vi "Sort Balls.vi"(11 "Detection Ball \nArray":T1[](array[typedef])) -> (3 "Sorted Detection Ball \nArray":T1[](array[typedef]))   [LabVIEW 2018]
uses:
  SSL Detection Ball.ctl
  <vilib>/Analysis/Matrix/Datatypes/RealMatrix.ctl
  <vilib>/Analysis/Matrix/NI_Matrix.lvlib
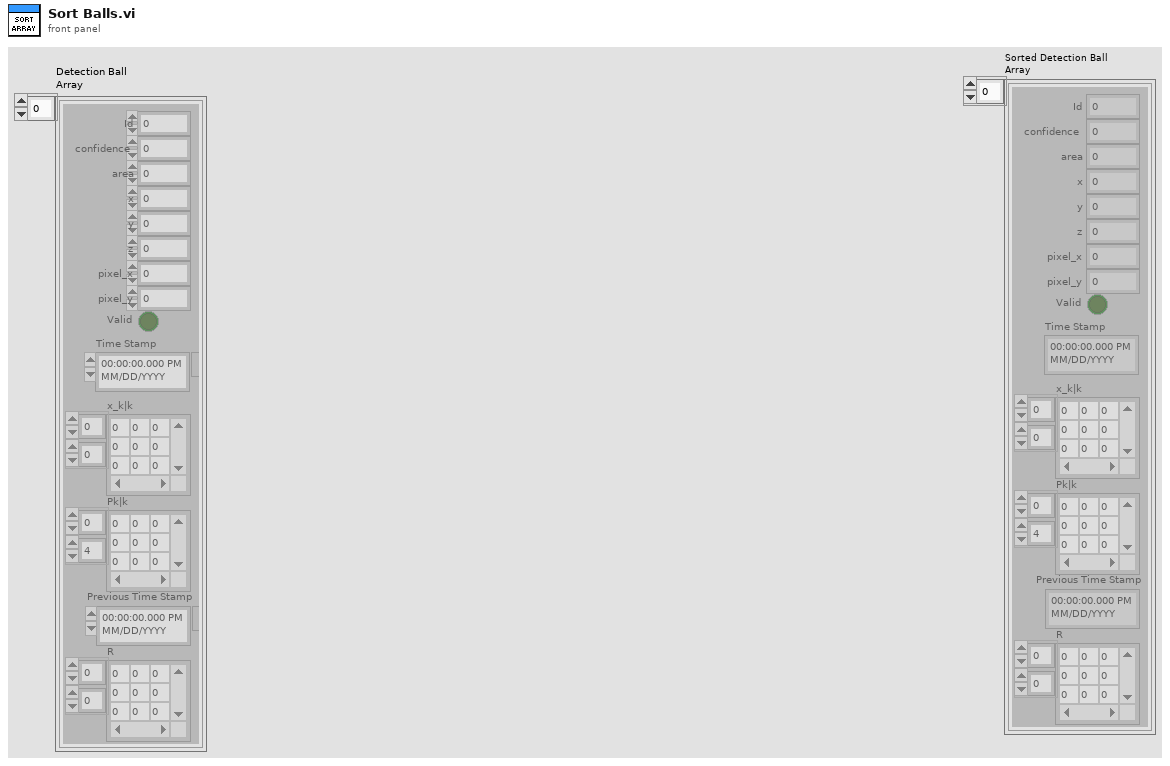
[diagram p1: front panel]
types:
  T1 = typedef "SSL Detection Ball.ctl" = cluster{"x":sgl, "area":u32, "confidence":sgl, "y":sgl, "z":sgl, "pixel_x":sgl, "pixel_y":sgl, "Valid":bool, "Time Stamp":timestamp, "x_k|k":T2, "Pk|k":T2, "Id":u32, "Previous Time Stamp":timestamp, "R":T2}
  T2 = typedef "NI_Matrix.lvlib/RealMatrix.ctl" = dbl[][]
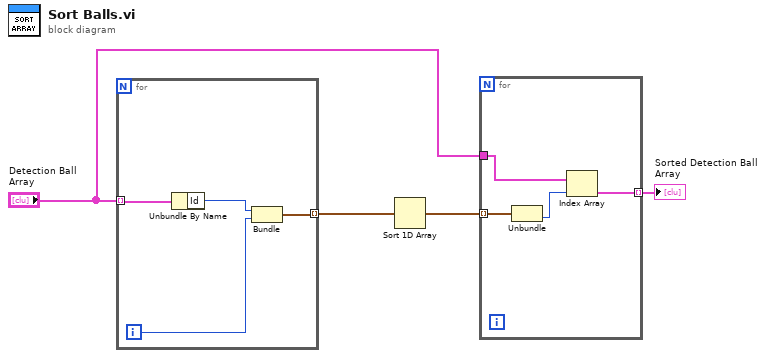
[diagram p0: block diagram]
diagram:
  n1 = for {
    tunnel: "Detection Ball \nArray" -> [w8] mode=indexing
    tunnel: [w5] -> w4 mode=indexing
    i -> [w6]
    n2 = Unbundle By Name(w8) -> ("Id"=w7:u32)
    n3 = Bundle("Id"=w7, w6) -> (w5:cluster{"Id":u32, i32})  [unwired: 1 in]
  }
  n4 = Sort 1D Array(array=w4) -> (sorted array=w3:cluster{"Id":u32, i32}[])
  n5 = for {
    tunnel: w3 -> [w11] mode=indexing
    tunnel: "Detection Ball \nArray" -> [w12]
    tunnel: [w9] -> w1 mode=indexing
    n6 = Unbundle(w11) -> (w10:i32)  [unwired: 1 out]
    n7 = Index Array(array=w12, index=w10) -> (element=w9:T1)
  }
  "Sorted Detection Ball \nArray" <- w1
